vi "Test - Draw Filled Triangle.vi"() -> ()   [LabVIEW 2020, in "Raster (FPGA).lvlib"]
uses:
  Raster (FPGA).lvlib
  Triangle.ctl
  Vertex.ctl
  Vector 3D.ctl
  UV.ctl
  Rectangle Dimensions.ctl
  Round Vertex.vi
  Calculate Line Reciprocal.vi
  Check Is Triangle Flat Bottomed.vi
  Round SGL.vi
  <vilib>/picture/picture.llb/Draw True-Color Pixmap.vi
panel:
  out "Numeric":i32
  out "new picture":picture
  in  "Triangle":T1={"Vertex 1"={"Position"={"x"=75.0, "y"=25.0, "z"=0.0}, "UV"={"u"=0.0, "v"=0.0}, "Colour"=12517256}, "Vertex 2"={"Position"={"x"=500.0, "y"=450.0, "z"=0.0}, "UV"={"u"=0.0, "v"=0.0}, "Colour"=12517256}, "Vertex 3"={"Position"={"x"=50.0, "y"=200.0, "z"=0.0}, "UV"={"u"=0.0, "v"=0.0}, "Colour"=12517256}, "Colour"=5308226} {"Vertex 3"."UV"."v" min=0 max=1 step=0.1; "Vertex 3"."UV"."u" min=0 max=1 step=0.1; "Vertex 2"."UV"."v" min=0 max=1 step=0.1; "Vertex 2"."UV"."u" min=0 max=1 step=0.1; "Vertex 1"."UV"."v" min=0 max=1 step=0.1; "Vertex 1"."UV"."u" min=0 max=1 step=0.1}
  # "(0,0)"
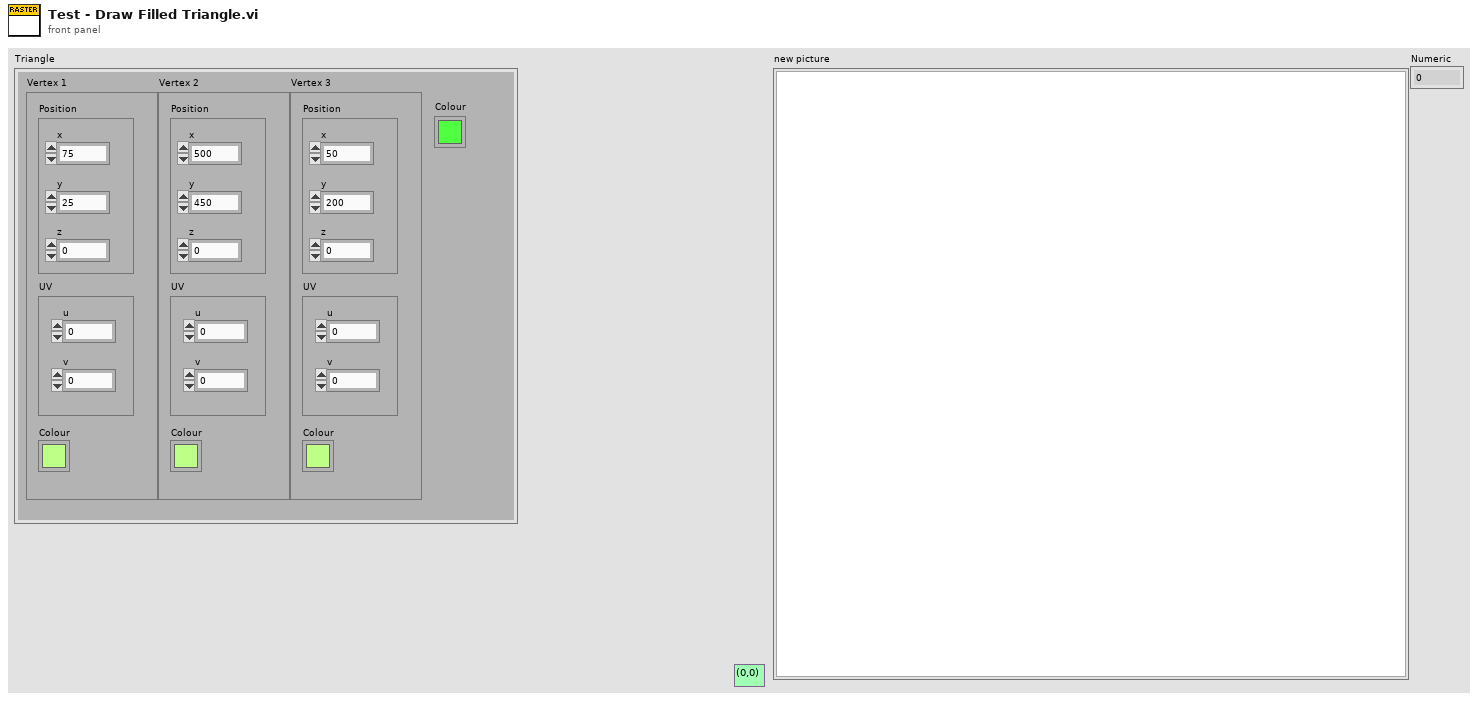
[diagram p1: front panel]
types:
  T1 = typedef "Raster (FPGA).lvlib/Triangle.ctl" = cluster{"Vertex 1":T2, "Vertex 2":T2, "Vertex 3":T2, "Colour":u32}
  T2 = typedef "Raster (FPGA).lvlib/Vertex.ctl" = cluster{"Position":T3, "UV":T4, "Colour":u32}
  T3 = typedef "Raster (FPGA).lvlib/Vector 3D.ctl" = cluster{"x":sgl, "y":sgl, "z":sgl}
  T4 = typedef "Raster (FPGA).lvlib/UV.ctl" = cluster{"u":sgl, "v":sgl}
  T5 = typedef "Raster (FPGA).lvlib/Rectangle Dimensions.ctl" = cluster{"Width":u32, "Height":u32}
  T6 = typedef "Raster (FPGA).lvlib/Triangle (Sorted).ctl" = cluster{"Top Vertex":T2, "Mid Vertex":T2, "Bottom Vertex":T2, "Colour":u32}
  T7 = typedef "Raster (FPGA).lvlib/Reciprocals.ctl" = cluster{"Bottom --> Top":sgl, "Bottom --> Middle":sgl, "Middle --> Top":sgl}
  T8 = typedef "Raster (FPGA).lvlib/Current Row.ctl" = cluster{"Start Column":sgl, "End Column":sgl}
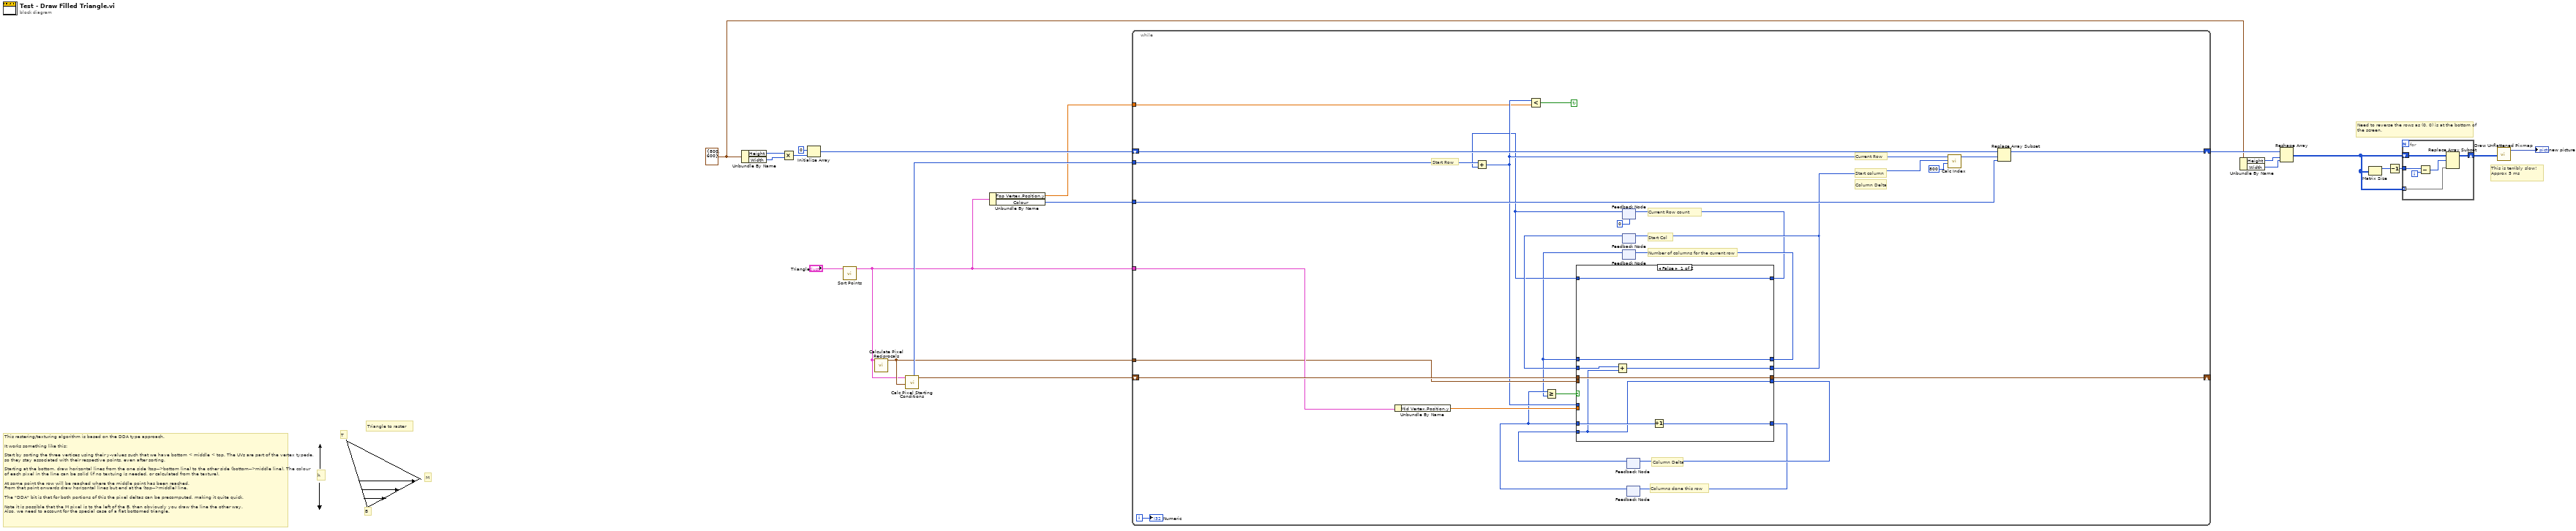
[diagram p0: block diagram]
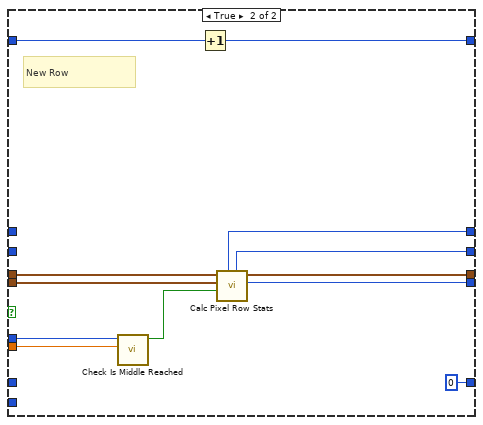
[diagram p2: hidden frame]
diagram:
  w12 = T5 {"Width"=800, "Height"=600} ("Screen Dimensions")
  # "h"
  # "Triangle to raster"
  # "M"
  # "T"
  # "B"
  # "This rastering/texturing algorithm is based on the DDA type approach.\n\nIt works something like this:\n\nStart by sorting the three vertices using their y-values such that we have bottom < middle < top. The UVs are part of the vertex typede, so they stay associated with their respective points, even after sorting.\n\nStarting at the bottom, draw horizontal lines from the one side (top-->bottom line) to the other side (bottom-->middle line). The colour of each pixel in the line can be solid (if no textuing is needed, or calculated from the texture).\n\nAt some point the row will be reached where the middle point has been reached.\nFrom that point onwards draw horizontal lines but end at the (top-->middle) line.\n\nThe \"DDA\" bit is that for both portions of this the pixel deltas can be precomputed, making it quite quick.\n\nNote it is possible that the M pixel is to the left of the B, then obviously you draw the line the other way.\nAlso, we need to account for the special case of a flat bottomed triangle."
  # "Need to reverse the rows as (0, 0) is at the bottom of the screen."
  # "This is terribly slow!\nApprox 5 ms"
  n1 = Unbundle By Name(w12) -> ("Height"=w11:u32, "Width"=w10:u32)
  n2 = Multiply(x=w11, y=w10) -> (x*y=w9:u32)
  n3 = Initialize Array(u32 0 ("element"), w9) -> (w8:u32[])
  n4 = call "Sort Points.vi"("Triangle"="Triangle") -> ("Sorted Triangle"=w2:T6)  [unwired: 10 in]
  n5 = call "Calculate Pixel Reciprocals.vi"("Sorted Triangle"=w2) -> ("Columns Pixels Per Row"=w4:T7)  [unwired: 10 in]
  n6 = call "Calc Pixel Starting Conditions.vi"("Reciprocals"=w4, "Sorted Vertices (V1 is top)"=w2) -> ("Start Row Columns"=w7:T8, "Start Row"=w6:i32)  [unwired: 8 in]
  n7 = Unbundle By Name(w2) -> ("Top Vertex.Position.y"=w1:sgl, "Colour"=w3:u32)
  n8 = while {
    shift-right: [w48] -> w19
    shift-left: w8 -> [w47]
    shift-right: [w44] -> _
    shift-left: w7 -> [w42]
    tunnel: w2 -> [w41]
    tunnel: w6 -> [w43]
    tunnel: w4 -> [w39]
    tunnel: w3 -> [w38]
    tunnel: w1 -> [w36]
    i -> [w40]
    stop <- w45 continue-if-true
    # "Columns done this row"
    # "Column Delta"
    # "Current Row count"
    # "Start Col"
    # "Number of columns for the current row"
    # "Column Delta"
    # "Current Row"
    # "Start column"
    # "Start Row"
    n9 = Unbundle By Name(w41) -> ("Mid Vertex.Position.y"=w46:sgl)
    n10 = feedback #1(0) -> (w28:i32)
    n11 = Add(x=w43, y=w28) -> (x+y=w37:i32)
    n12 = Less?(x=w37, y=w36) -> (x < y?=w45:bool)
    n13 = feedback #2() -> (w33:i32)  [unwired: 1 in]
    n14 = feedback #3() -> (w25:i32)  [unwired: 1 in]
    n15 = feedback #4() -> (w31:i32)  [unwired: 1 in]
    n16 = feedback #5() -> (w26:i32)  [unwired: 1 in]
    n17 = Greater Or Equal?(x=w26, y=w25) -> (x >= y?=w24:bool)
    n18 = case shown="False" w24 {
      tunnel: w46 -> [_ w68]
      tunnel: [w55 w67] -> w44
      tunnel: w42 -> [w55 w66]
      tunnel: w39 -> [_ w65]
      tunnel: [w56 w64] -> w35
      tunnel: [w49 w62] -> w32
      tunnel: [w50 w61] -> w34
      tunnel: w37 -> [_ w60]
      tunnel: w25 -> [w56 _]
      tunnel: w33 -> [w51 _]
      tunnel: w31 -> [w49 _]
      tunnel: w28 -> [w54 w59]
      tunnel: [w54 w58] -> w29
      tunnel: [w52 0] -> w27
      tunnel: w26 -> [w53 _]
      frame False {
        n19 = Add(x=w51, y=w49) -> (x+y=w50:i32)
        n20 = Increment(x=w53) -> (x+1=w52:i32)
      }
      frame True {
        # "New Row"
        n21 = call "Check Is Middle Reached.vi"("Middle y"=w68, "Current Row"=w60) -> ("Reached Middle"=w63:bool)  [unwired: 9 in]
        n22 = Increment(x=w59) -> (x+1=w58:i32)
        n23 = call "Calc Pixel Row Stats.vi"("Reached Middle"=w63, "Reciprocals"=w65, "Current Row"=w66) -> ("Column Delta"=w62:i32, "Next Row"=w67:T8, "Start Col"=w61:i32, "Number Of Cols This Row"=w64:i32)  [unwired: 4 in, 1 out]
      }
    }
    n24 = feedback-in #1(w29) -> ()
    n25 = feedback-in #2(w34) -> ()
    n26 = feedback-in #3(w35) -> ()
    n27 = feedback-in #4(w32) -> ()
    n28 = feedback-in #5(w27) -> ()
    n29 = call "Calc Index.vi"("Cols Per Row"=800, "Col"=w34, "Row"=w37) -> ("Index"=w22:i32)  [unwired: 8 in]
    n30 = Replace Array Subset(array=w47, new element=w38, index=w22) -> (w48:u32[])
    "Numeric" <- w40
  }
  n31 = Unbundle By Name(w12) -> ("Height"=w21:u32, "Width"=w20:u32)
  n32 = Reshape Array(w19, w21, w20) -> (w15:u32[][])
  n33 = Matrix Size(0:w15) -> (1:w17:i32)  [unwired: 1 out]
  n34 = Decrement(x=w17) -> (x-1=w16:i32)
  n35 = for {
    tunnel: w15 -> [w70] mode=indexing
    shift-right: [w69] -> w18
    shift-left: w15 -> [w74]
    tunnel: w16 -> [w73]
    i -> [w72]
    n36 = Subtract(x=w73, y=w72) -> (x-y=w71:i32)
    n37 = Replace Array Subset(array=w74, new element=w70, index (row)=w71) -> (w69:u32[][])  [unwired: 1 in]
  }
  n38 = call-poly <vilib>:"Draw Unflattened Pixmap.vi"("data (RGB format)"=w18) -> ("new picture"=→"new picture":picture)  [unwired: 8 in]
